vi "EditorSub saveAsData.vi"(8 "error in (no error)":errorcluster, 9 "exportData":T1) -> (0 "error out":errorcluster)   [LabVIEW 2018]
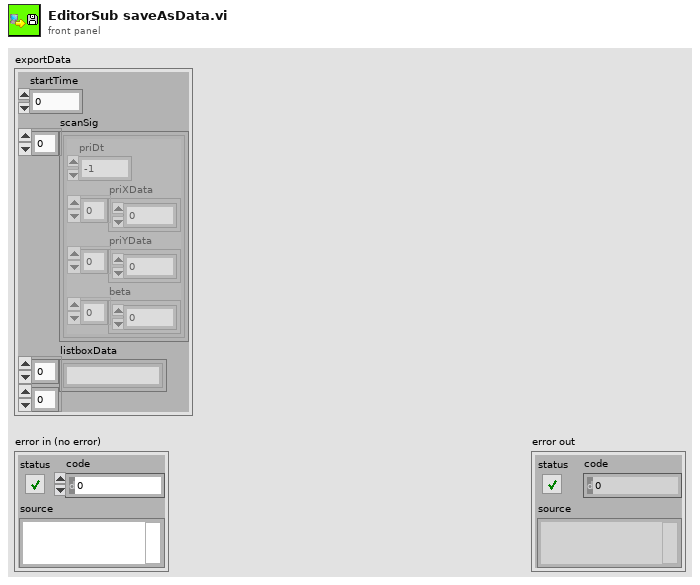
[diagram p1: front panel]
types:
  T1 = cluster{"startTime":dbl, "scanSig":cluster{"priDt":dbl, "priXData":dbl[], "priYData":sgl[], "beta":dbl[]}[], "listboxData":string[][]}
  T2 = enum16{"open", "replace", "create", "open or create", "replace or create", "replace or create with confirmation"}
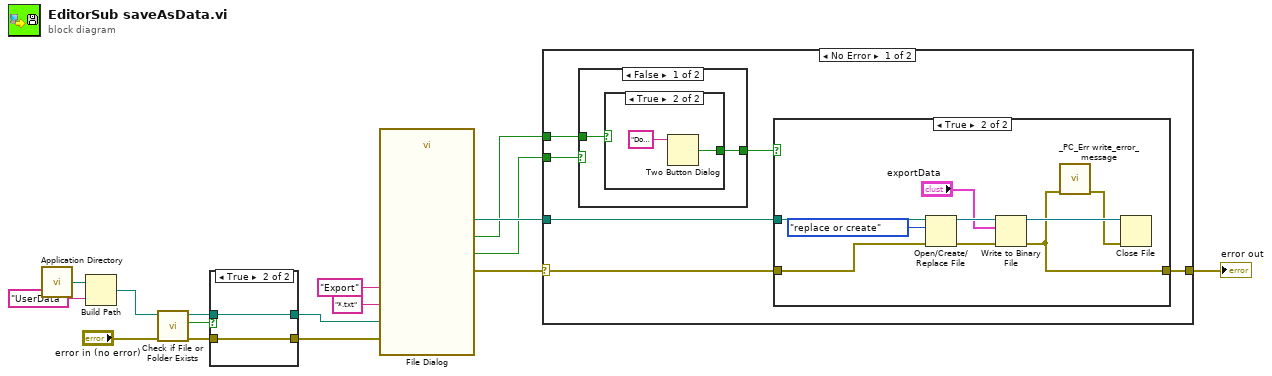
[diagram p0: block diagram]
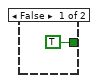
[diagram p2: hidden frame]
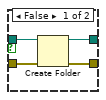
[diagram p6: hidden frame]
diagram:
  n1 = call <vilib>:"Application Directory.vi"() -> ("Application Directory"=w16:path)
  n2 = Build Path(base path=w16, name or relative path="UserData") -> (appended path=w14:path)
  n3 = call <vilib>:"Check if File or Folder Exists.vi"("error in (no error)"="error in (no error)", "path"=w14) -> ("error out"=w11:errorcluster, "file or folder exists?"=w12:bool, "dup path"=w13:path)  [unwired: 7 in]
  n4 = case shown="True" w12 {
    tunnel: w13 -> [w20 w22]
    tunnel: w11 -> [w19 w21]
    tunnel: [w18 w22] -> w10
    tunnel: [w17 w21] -> w6
    frame False {
      n5 = Create Folder(path (use dialog)=w20, error in=w19) -> (created path=w18:path, error out=w17:errorcluster)  [unwired: 1 in, 1 out]
    }
    frame True {
    }
  }
  n6 = call "File Dialog"("start path"=w10, "default name"="Export", "error in"=w6, "pattern (all files)"="*.txt") -> ("selected path"=w7:path, "exists"=w5:bool, "cancelled"=w4:bool, "error out"=w3:errorcluster)  [unwired: 8 in]
  n7 = case shown="No Error" w3 {
    selector: w3 -> [w24 w44]
    tunnel: w7 -> [w28 _]
    tunnel: w5 -> [w27 _]
    tunnel: w4 -> [w26 _]
    tunnel: [w23 w44] -> w2
    frame No Error {
      n8 = case shown="False" w26 {
        tunnel: w27 -> [w30 _]
        tunnel: [w29 _] -> w25
        frame False {
          n9 = case shown="True" w30 {
            tunnel: [TRUE ("T button?") w32] -> w29
            frame False {
            }
            frame True {
              n10 = Two Button Dialog(message="Do you want to overwrite this file?") -> (T button?=w32:bool)  [unwired: 2 in]
            }
          }
        }
        frame True {
        }
      }
      n11 = case shown="True" w25 {
        tunnel: w28 -> [_ w43]
        tunnel: w24 -> [w34 w42]
        tunnel: [w34 w35] -> w23
        frame False {
        }
        frame True {
          n12 = Open/Create/Replace File(file path (use dialog)=w43, error in=w42, operation (0:open)=T2."replace or create") -> (refnum out=w41:refnum<file>, error out=w39:errorcluster)  [unwired: 3 in, 1 out]
          n13 = Write to Binary File(file (use dialog)=w41, data="exportData", error in=w39) -> (refnum out=w37:refnum<file>, error out=w35:errorcluster)  [unwired: 3 in, 1 out]
          n14 = call "_PC_Err write_error_message.vi"("error in"=w35) -> ("error out"=w36:errorcluster)  [unwired: 10 in]
          n15 = Close File(refnum=w37, error in=w36) -> ()  [unwired: 2 out]
        }
      }
    }
    frame Error {
    }
  }
  "error out" <- w2
